vi "Decode MHTML Base64.vi"(7 "Encoded String\n(Base64)":string) -> (8 "Decoded Binary\nString":string)   [LabVIEW 2011]
panel:
  out "Array Constant":u8[](array[numeric])
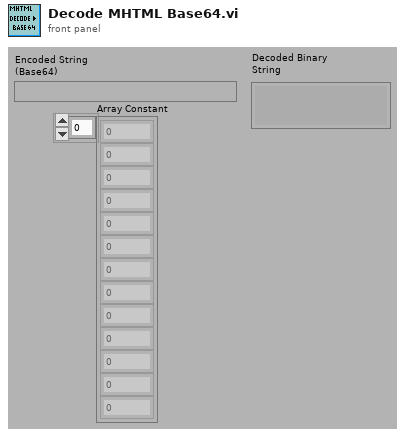
[diagram p1: front panel]
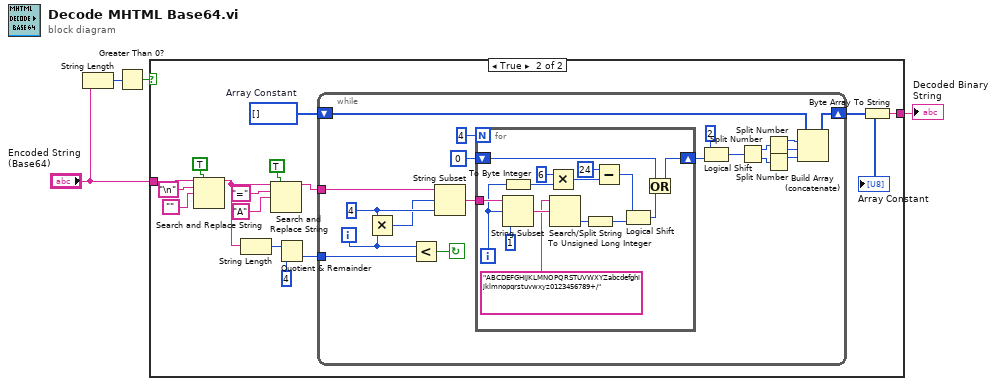
[diagram p0: block diagram]
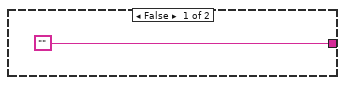
[diagram p2: hidden frame]
diagram:
  n1 = String Length(string="Encoded String\n(Base64)") -> (length=w4:i32)
  n2 = Greater Than 0?(x=w4) -> (x > 0?=w3:bool)
  n3 = case shown="True" w3 {
    tunnel: "Encoded String\n(Base64)" -> [_ w17]
    tunnel: ["" w8] -> w1
    frame False {
    }
    frame True {
      w10 = u8[] []  # Array Constant
      n4 = Search and Replace String(replace all?=TRUE, input string=w17, search string="\n", replace string="") -> (result string=w6:string)  [unwired: 1 in, 6 out]
      n5 = String Length(string=w6) -> (length=w13:i32)
      n6 = Search and Replace String(replace all?=TRUE, input string=w6, search string="=", replace string="A") -> (result string=w7:string)  [unwired: 1 in, 6 out]
      n7 = Quotient & Remainder(x=w13, y=4 ("length (rest)")) -> (floor(x/y)=w11:i32)  [unwired: 1 out]
      n8 = while {
        shift-left: w10 -> [w25]
        shift-right: [w24] -> w9
        tunnel: w7 -> [w37]
        tunnel: w11 -> [w39]
        i -> [w23]
        stop <- w38 continue-if-true
        w22 = 4 ("length (rest)")
        n9 = Multiply(x=w22, y=w23) -> (x*y=w21:i32)
        n10 = Less?(x=w23, y=w39) -> (x < y?=w38:bool)
        n11 = String Subset(string=w37, offset (0)=w21, length (rest)=w22) -> (substring=w26:string)
        n12 = for {
          N: 4 -> [_]
          tunnel: w26 -> [w50]
          shift-right: [w43] -> w29
          shift-left: u32 0 ("y") -> [w49]
          i -> [w45]
          n13 = To Byte Integer(number=w45) -> (8bit integer=w41:i8)
          n14 = String Subset(string=w50, offset (0)=w45, length (rest)=1 ("length")) -> (substring=w53:string)
          n15 = Multiply(x=i8 6 ("y"), y=w41) -> (x*y=w46:i8)
          n16 = Search/Split String(string="ABCDEFGHIJKLMNOPQRSTUVWXYZabcdefghijklmnopqrstuvwxyz0123456789+/", search string/char (-)=w53) -> (offset of match=w51:i32)  [unwired: 3 out]
          n17 = To Unsigned Long Integer(number=w51) -> (unsigned 32bit integer=w42:u32)
          n18 = Subtract(x=i8 24 ("y"), y=w46) -> (x-y=w44:i8)
          n19 = Logical Shift(y=w44, x=w42) -> (x << y=w40:u32)
          n20 = Or(x=w49, y=w40) -> (x .or. y?=w43:u32)
        }
        n21 = Logical Shift(y=i8 2, x=w29) -> (x << y=w28:u32)
        n22 = Split Number(x=w28) -> (hi(x)=w35:u16, lo(x)=w34:u16)
        n23 = Split Number(x=w35) -> (hi(x)=w33:u8, lo(x)=w32:u8)
        n24 = Split Number(x=w34) -> (hi(x)=w31:u8)  [unwired: 1 out]
        n25 = Build Array (concatenate)(w25, w33, w32, w31) -> (w24:u8[])
      }
      "Array Constant" <- w9
      n26 = Byte Array To String(unsigned byte array=w9) -> (string=w8:string)
    }
  }
  "Decoded Binary\nString" <- w1
